vi "Initialization VI.vi"(8 "error in (no error)":errorcluster, 10 "Custom XML":string, 11 "Device Item Ref in":T1 format="%.0x") -> (0 "error out":errorcluster, 3 "Device Item Ref out":T1 format="%.0x")   [LabVIEW 2021, in "G5 Regatron Custom Device System Explorer.lvlib"]
uses:
  G5 Regatron Custom Device System Explorer.lvlib
  <vilib>/NI VeriStand/Custom Device API/Custom Device Item Ref.ctl
  <vilib>/NI/NI VeriStand Custom Device Import and Export Tool/ImportExport.lvlib
  <vilib>/NI VeriStand/Custom Device API/Custom Device API.lvlib
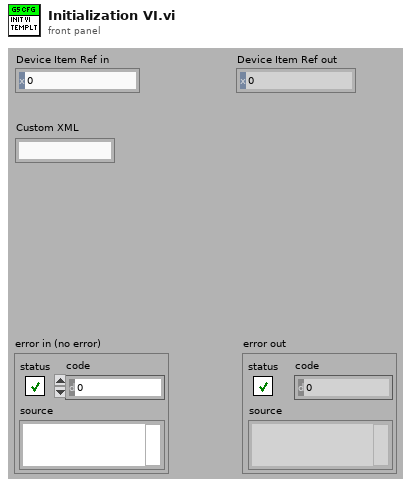
[diagram p1: front panel]
types:
  T1 = typedef "Custom Device API.lvlib/Custom Device Item Ref.ctl" = u64
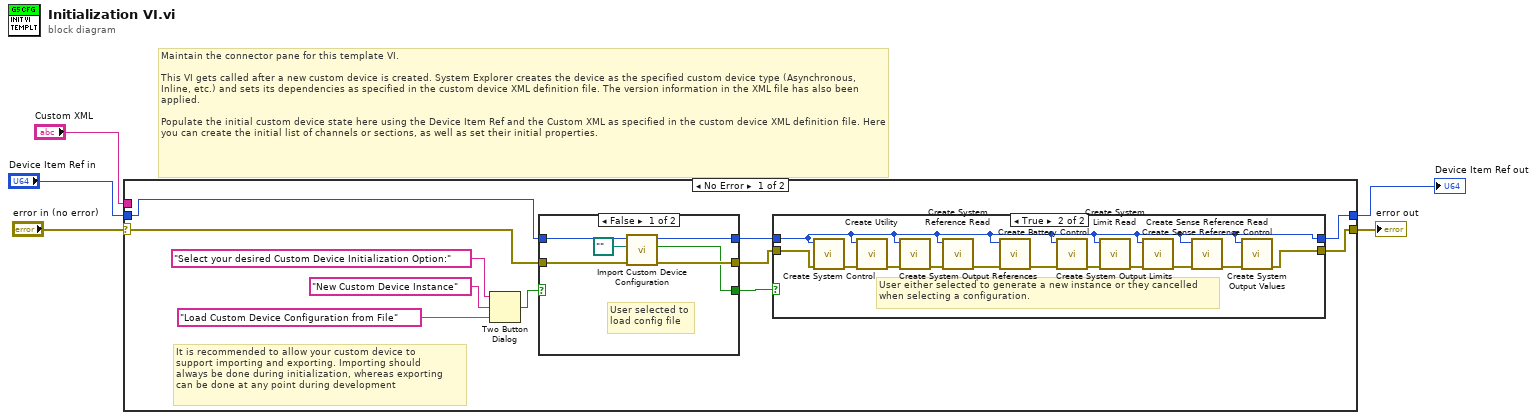
[diagram p0: block diagram]
diagram:
  # "Maintain the connector pane for this template VI.\n\nThis VI gets called after a new custom device is created. System Explorer creates the device as the specified custom device type (Asynchronous, Inline, etc.) and sets its dependencies as specified in the custom device XML definition file. The version information in the XML file has also been applied.\n\nPopulate the initial custom device state here using the Device Item Ref and the Custom XML as specified in the custom device XML definition file. Here you can create the initial list of channels or sections, as well as set their initial properties."
  n1 = case shown="No Error" "error in (no error)" {
    selector: "error in (no error)" -> [w11 w41]
    tunnel: [w6 w41] -> w5
    tunnel: [w7 w40] -> w3
    tunnel: "Device Item Ref in" -> [w12 w40]
    tunnel: "Custom XML" -> [_ _]
    frame No Error {
      # "It is recommended to allow your custom device to\nsupport importing and exporting. Importing should\nalways be done during initialization, whereas exporting\ncan be done at any point during development"
      n2 = Two Button Dialog(message="Select your desired Custom Device Initialization Option:", 1:"Load Custom Device Configuration from File" ("F button name (\"Cancel\")"), 2:"New Custom Device Instance" ("T button name (\"OK\")")) -> (T button?=w13:bool)
      n3 = case shown="False" w13 {
        selector: w13 -> [_ w37]
        tunnel: w12 -> [w36 w39]
        tunnel: [w35 w39] -> w8
        tunnel: w11 -> [w33 w38]
        tunnel: [w32 w38] -> w10
        tunnel: [w31 w37] -> w9
        frame False {
          # "User selected to\nload config file"
          n4 = call <vilib>:"Import Custom Device Configuration.vi"("error in (no error)"=w33, "Path"=path "", "NodeID"=w36) -> ("error out"=w32:errorcluster, "cancelled"=w31:bool, "NodeID out"=w35:u64)  [unwired: 6 in]
        }
        frame True {
          # "User selected new\ncustom device. Do\nnothing in this case\nand handle new\ngeneration in the\nnext case structure"
        }
      }
      n5 = case shown="True" w9 {
        tunnel: w8 -> [w18 w19]
        tunnel: w10 -> [w17 w30]
        tunnel: [w17 w21] -> w6
        tunnel: [w18 w19] -> w7
        frame False {
          # "User selected to import from configuration and didn't cancel import"
        }
        frame True {
          # "User either selected to generate a new instance or they cancelled\nwhen selecting a configuration."
          n6 = call "Create System Control.vi"("error in (no error)"=w30, "Device Item Ref in"=w19) -> ("error out"=w27:errorcluster)  [unwired: 9 in]
          n7 = call "Create Utility.vi"("error in (no error)"=w27, "Device Item Ref in"=w19) -> ("error out"=w23:errorcluster)  [unwired: 9 in]
          n8 = call "Create System Output References.vi"("error in (no error)"=w23, "Device Item Ref in"=w19) -> ("error out"=w29:errorcluster)  [unwired: 9 in]
          n9 = call "Create System Reference Read.vi"("error in (no error)"=w29, "Device Item Ref in"=w19) -> ("error out"=w28:errorcluster)  [unwired: 9 in]
          n10 = call "Create Battery Control.vi"("error in (no error)"=w28, "Device Item Ref in"=w19) -> ("error out"=w20:errorcluster)  [unwired: 9 in]
          n11 = call "Create System Output Limits.vi"("error in (no error)"=w20, "Device Item Ref in"=w19) -> ("error out"=w26:errorcluster)  [unwired: 9 in]
          n12 = call "Create System Limit Read.vi"("error in (no error)"=w26, "Device Item Ref in"=w19) -> ("error out"=w25:errorcluster)  [unwired: 9 in]
          n13 = call "Create Sense Reference Control.vi"("error in (no error)"=w25, "Device Item Ref in"=w19) -> ("error out"=w24:errorcluster)  [unwired: 9 in]
          n14 = call "Create Sense Reference Read.vi"("error in (no error)"=w24, "Device Item Ref in"=w19) -> ("error out"=w22:errorcluster)  [unwired: 9 in]
          n15 = call "Create System Output Values.vi"("error in (no error)"=w22, "Device Item Ref in"=w19) -> ("error out"=w21:errorcluster)  [unwired: 9 in]
        }
      }
    }
    frame Error {
    }
  }
  "error out" <- w5
  "Device Item Ref out" <- w3
